vi "mature_track.vi"(3 "Centerline Positions (Camera Pixel)":sgl[][][](array[numeric]), 4 "Track Centroid Positions (Camera Pixel)":sgl[][](array[numeric]), 5 "Within Track Index":i32) -> (0 "Corrrected Centerline Positions":sgl[][][](array[numeric]), 1 "head/tail flip":bool)   [LabVIEW 2019]
uses:
  euclidean_distance_single.vi
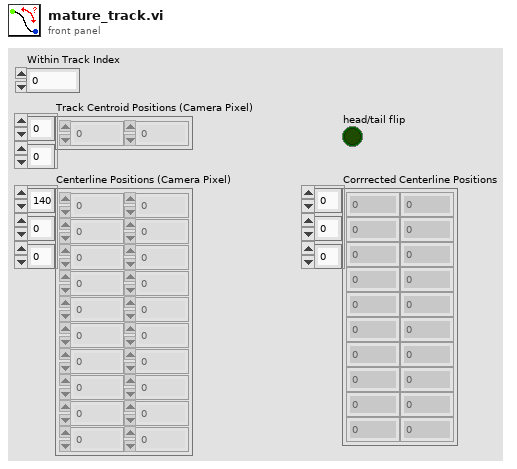
[diagram p1: front panel]
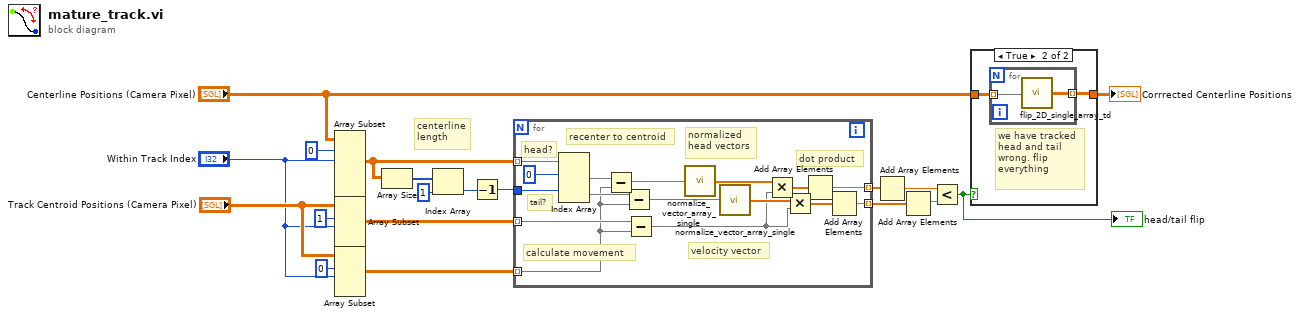
[diagram p0: block diagram]
diagram:
  # "centerline\nlength"
  n1 = Array Subset(array="Centerline Positions (Camera Pixel)", index (dim 0)=0 ("index (page)"), length (dim 0)="Within Track Index") -> (w19:sgl[][][])  [unwired: 4 in]
  n2 = Array Subset(array="Track Centroid Positions (Camera Pixel)", index (row)=1, length (row)="Within Track Index") -> (w5:sgl[][])  [unwired: 2 in]
  n3 = Array Subset(array="Track Centroid Positions (Camera Pixel)", index (row)=0, length (row)="Within Track Index") -> (w2:sgl[][])  [unwired: 2 in]
  n4 = Array Size(array=w19) -> (size(s)=w18:i32[])
  n5 = Index Array(array=w18, index=1) -> (element=w9:i32)
  n6 = Decrement(x=w9) -> (x-1=w8:i32)
  n7 = for {
    tunnel: w19 -> [w35] mode=indexing
    tunnel: w8 -> [w33]
    tunnel: w2 -> [w29] mode=indexing
    tunnel: w5 -> [w30] mode=indexing
    tunnel: [w22] -> w16 mode=indexing
    tunnel: [w21] -> w15 mode=indexing
    # "velocity vector"
    # "calculate movement"
    # "normalized\nhead vectors"
    # "dot product"
    # "recenter to centroid"
    # "tail?"
    # "head?"
    n8 = Index Array(array=w35, index (row) #1=0 ("index (row)"), index (row) #2=w33) -> (element #1=w32:sgl[], element #2=w31:sgl[])  [unwired: 2 in]
    n9 = Subtract(x=w32, y=w29) -> (x-y=w24:sgl[])
    n10 = Subtract(x=w31, y=w29) -> (x-y=w26:sgl[])
    n11 = Subtract(x=w30, y=w29) -> (x-y=w20:sgl[])
    n12 = call "normalize_vector_array_single.vi"("2 element vector"=w24) -> ("normalized vector out"=w23:sgl[])
    n13 = call "normalize_vector_array_single.vi"("2 element vector"=w26) -> ("normalized vector out"=w25:sgl[])
    n14 = Multiply(x=w23, y=w20) -> (x*y=w28:sgl[])
    n15 = Multiply(x=w25, y=w20) -> (x*y=w27:sgl[])
    n16 = Add Array Elements(numeric array=w28) -> (sum=w22:sgl)
    n17 = Add Array Elements(numeric array=w27) -> (sum=w21:sgl)
  }
  n18 = Add Array Elements(numeric array=w16) -> (sum=w14:sgl)
  n19 = Add Array Elements(numeric array=w15) -> (sum=w13:sgl)
  n20 = Less?(x=w14, y=w13) -> (x < y?=w11:bool)
  "head/tail flip" <- w11
  n21 = case shown="True" w11 {
    tunnel: "Centerline Positions (Camera Pixel)" -> [w36 w38]
    tunnel: [w36 w37] -> w10
    frame False {
      # "no flip required"
    }
    frame True {
      # "we have tracked\nhead and tail\nwrong. flip \neverything"
      n22 = for {
        tunnel: w38 -> [w40] mode=indexing
        tunnel: [w39] -> w37 mode=indexing
        n23 = call "flip_2D_single_array_td.vi"("Centerline"=w40) -> ("Array Flipped Top Down"=w39:sgl[][])
      }
    }
  }
  "Corrrected Centerline Positions" <- w10
